vi "GetControlRef.vi"(0 "VI Reference In":refnum<vi>, 7 "Control Path":string[](array[string]), 11 "error In":errorcluster) -> (4 "VI Reference Out":refnum<vi>, 8 "Ctl Refnum":refnum<vi>, 15 "error out":errorcluster)   [LabVIEW 2016]
doc: "<b>Gives the reference of controls in other VI.</b>\n\nThe path of the control should be given in the successive index of the array"
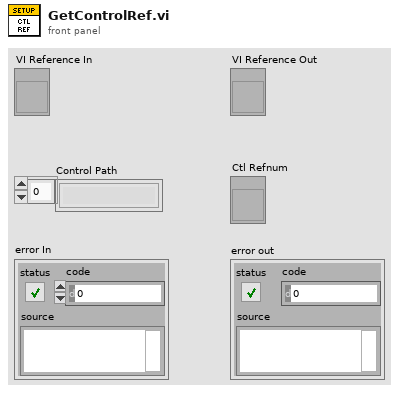
[diagram p1: front panel]
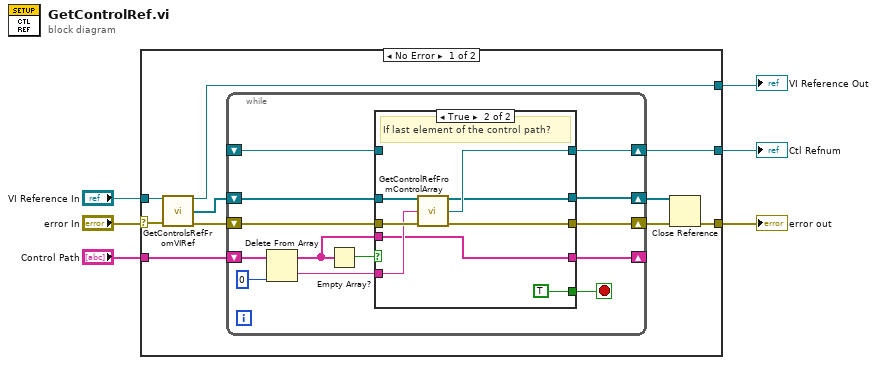
[diagram p0: block diagram]
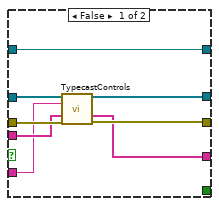
[diagram p2: hidden frame]
diagram:
  n1 = case shown="No Error" "error In" {
    selector: "error In" -> [w9 w47]
    tunnel: "Control Path" -> [w15 _]
    tunnel: [w8 w47] -> w5
    tunnel: [w12 _] -> w4
    tunnel: "VI Reference In" -> [w10 w46]
    tunnel: [w7 w46] -> w1
    frame No Error {
      n2 = call "GetControlsRefFromVIRef.vi"("VI Reference In"=w10, "Error In"=w9) -> ("VI Reference Out"=w7:refnum<vi>, "Controls[]"=w14:refnum<vi>[], "Error Out"=w11:errorcluster)  [unwired: 11 in]
      n3 = while {
        shift-right: [w25] -> w16
        shift-left: w11 -> [w26]
        shift-right: [w21] -> w13
        shift-left: w14 -> [w23]
        shift-right: [w22] -> w12
        shift-left: _ -> [w20]
        shift-right: [w17] -> _
        shift-left: w15 -> [w24]
        stop <- w19 stop-if-true
        n4 = Delete From Array(array=w24, index=0) -> (deleted portion=w27:string, array with subset deleted=w18:string[])  [unwired: 1 in]
        n5 = Empty Array?(array=w18) -> (empty?=w28:bool)
        n6 = case shown="True" w28 {
          tunnel: w23 -> [w37 w43]
          tunnel: w27 -> [w30 w44]
          tunnel: [w33 w41] -> w22
          tunnel: w26 -> [w36 w45]
          tunnel: [w34 w42] -> w25
          tunnel: [w35 w40] -> w21
          tunnel: w20 -> [w33 _]
          tunnel: [_ TRUE] -> w19
          tunnel: w18 -> [w32 w38]
          tunnel: [w31 w38] -> w17
          frame False {
            n7 = call "TypecastControls.vi"("Controls[]"=w37, "Control Name"=w30, "Control Path In"=w32, "error In"=w36) -> ("Sub Controls[]"=w35:refnum<vi>[], "Control Path Out"=w31:string[], "error out"=w34:errorcluster)  [unwired: 9 in]
          }
          frame True {
            # "If last element of the control path?"
            n8 = call "GetControlRefFromControlArray.vi"("Controls[]"=w43, "Control Name"=w44, "error In"=w45) -> ("Remaining Controls[]"=w40:refnum<vi>[], "Target Control"=w41:refnum<vi>, "error out"=w42:errorcluster)  [unwired: 10 in]
          }
        }
      }
      n9 = Close Reference(reference=w13, error in (no error)=w16) -> (error out=w8:errorcluster)
    }
    frame Error {
    }
  }
  "Ctl Refnum" <- w4
  "error out" <- w5
  "VI Reference Out" <- w1
